vi "[CS] Main.vi"() -> ()   [LabVIEW 2014]
uses:
  NI Vision Camera Device/NI Vision Camera Device.lvclass
  NI Vision Camera Device/Configuration.ctl
panel:
  in  "Camera:Gain":dbl caption="Gain" min=0.0 max=20.0
  in  "Camera:Exposure":dbl=1000.0 caption="Exposure (µs)" min=20.0 max=1000000.0
  out "Camera":refnum<class "NI Vision Camera Device.lvclass">
  out "Camera:SizeY":u32=1040
  out "Camera:SizeX":u32=1392
  out "Avg":dbl[][](graph)
  out "Camera:FrameCount":u64
  out "Realtime":u16[][](graph)
  out "Exp:Progress":dbl(slide)=1.0 scale=0.0..1.0
  in  "Exp:MaxCount":u64=100
  in  "Exp:Start":bool
  in  "Exp:Cont":bool
  in  "Exp:Abort":bool
  in  "Camera:Threshold":u16=5 caption="Threshold"
  in  "Exp:Save":bool
  in  "Suffix":string
  in  "Camera:Start":bool
  in  "Camera:Stop":bool
  in  "Exp:Count":u64=100
  out "App:Basepath":path=path "C:/Users/mpdlab/Desktop/CameraSoftware/data"
  out "Camera:Sum":u64[][](array[numeric])
  out "App:Exit":bool
  out "Camera:Status":bool=TRUE
  # "Experiment"
  # "Camera"
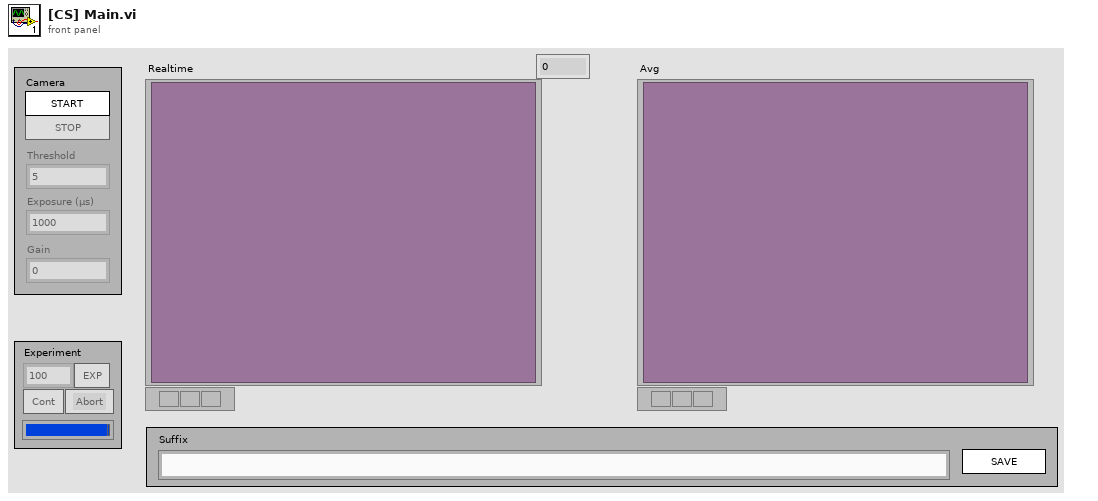
[diagram p1: front panel]
types:
  T1 = enum8{"Enabled", "Disabled", "Disabled and Grayed Out"}
  T2 = enum32{"invalid app kind", "Development System", "Run Time System", "Student Edition", "Embedded LabVIEW", "Evaluation", "Custom"}
  T3 = enum32{"Invalid", "Standard", "Closed", "Hidden", "Minimized", "Maximized"}
  T4 = typedef "NI Vision Camera Device.lvclass/Configuration.ctl" = cluster{"Exposure":dbl, "Gain":dbl}
  T5 = cluster{"Core":cluster{"Current VI Reference":refnum<vi>, "Close Panel on Exit?":bool}, "Camera:Status":bool}
  T6 = cluster{"Current VI Reference":refnum<vi>, "Close Panel on Exit?":bool}
  T7 = typedef "imagedata.ctl" = cluster{"image type":i32, "image depth":i32, "image":u8[], "mask":u8[], "colors":u32[], "Rectangle":cluster{"left":i16, "top":i16, "right":i16, "bottom":i16}}
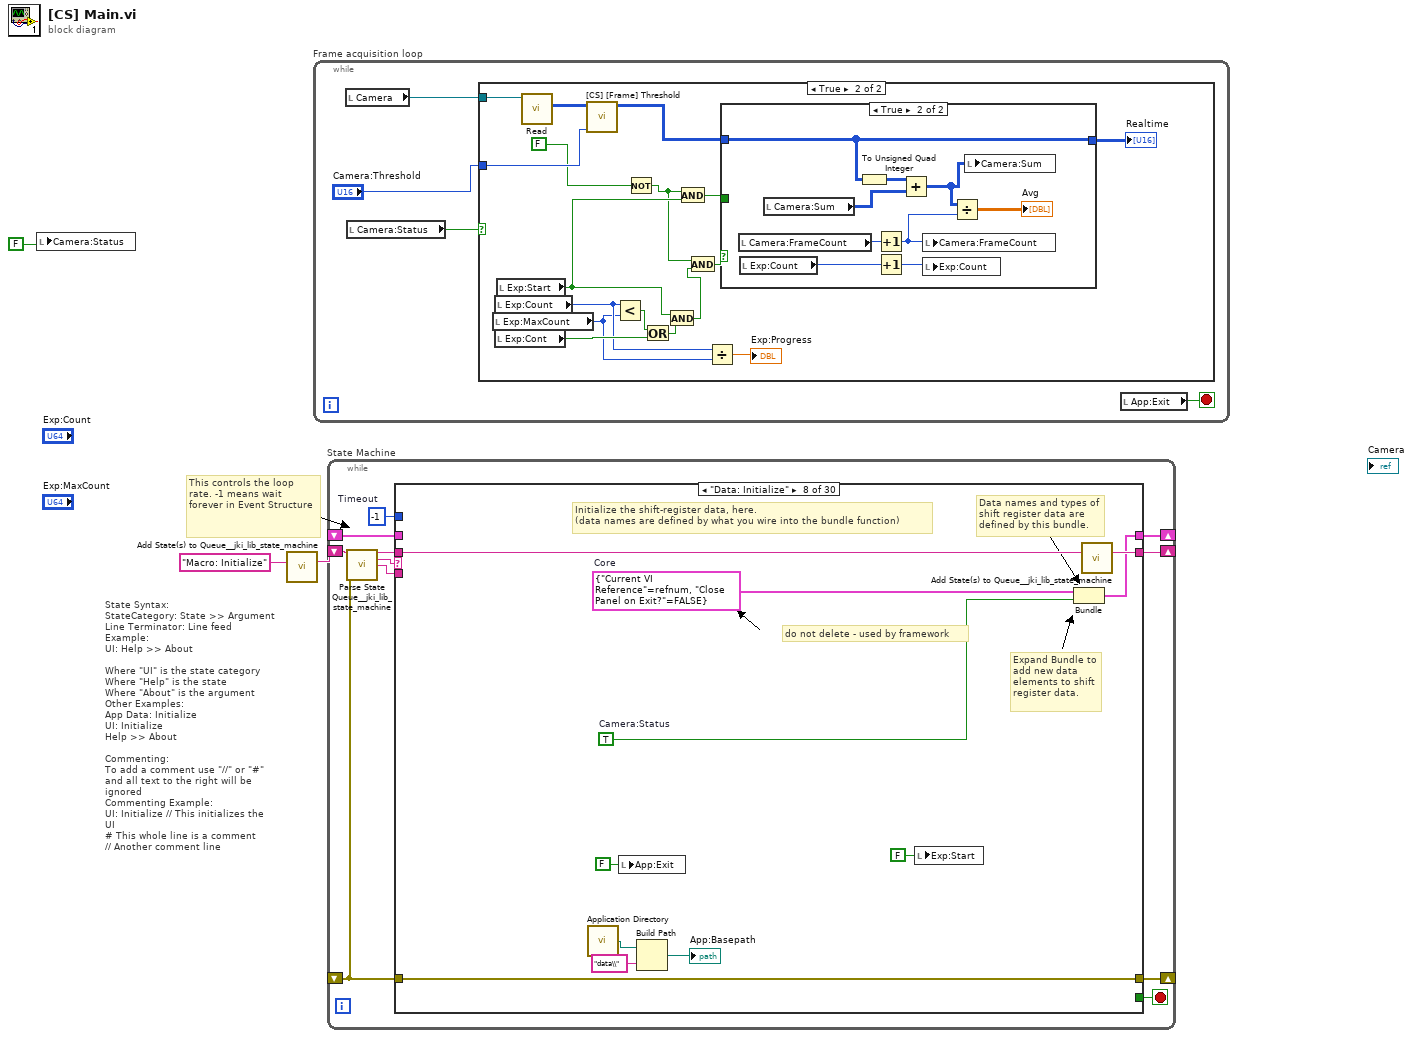
[diagram p0: block diagram]
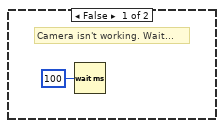
[diagram p2: hidden frame]
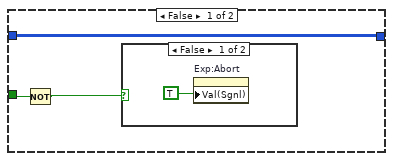
[diagram p3: hidden frame]
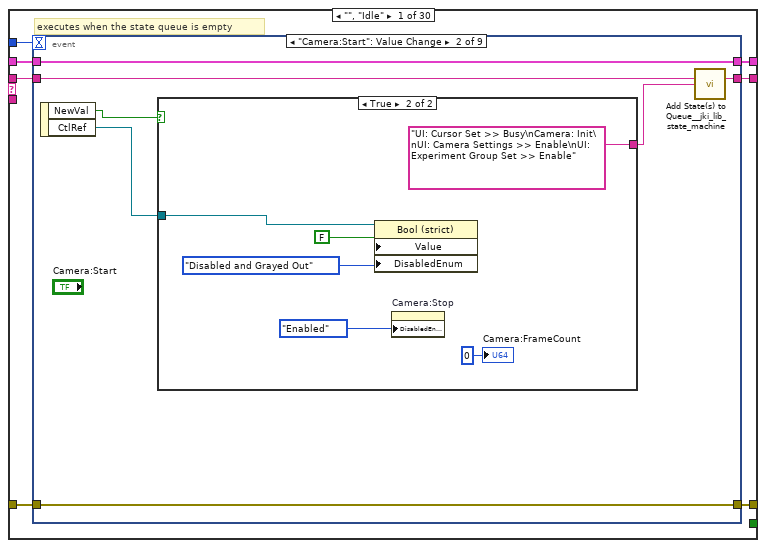
[diagram p5: hidden frame]
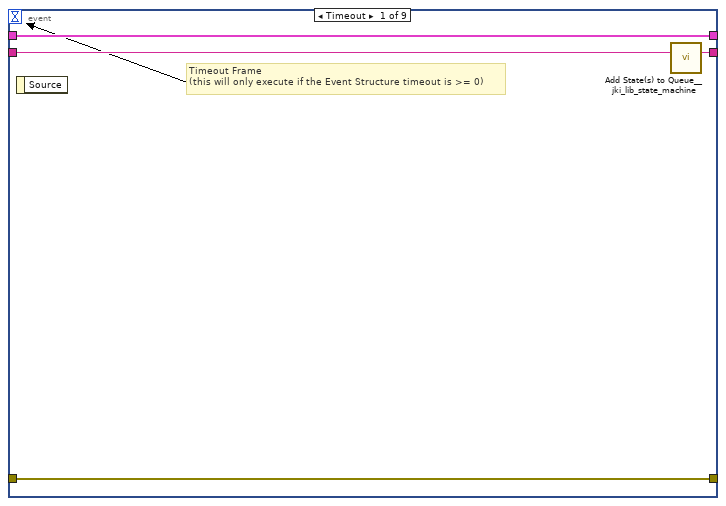
[diagram p6: hidden frame]
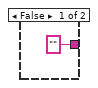
[diagram p7: hidden frame]
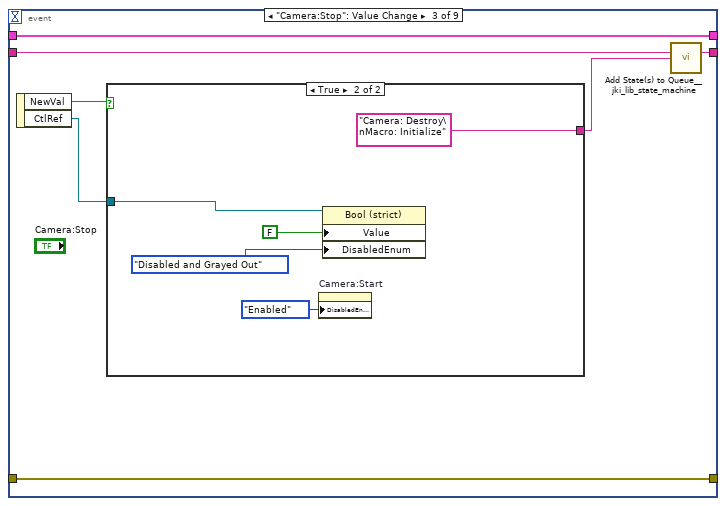
[diagram p8: hidden frame]
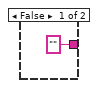
[diagram p9: hidden frame]
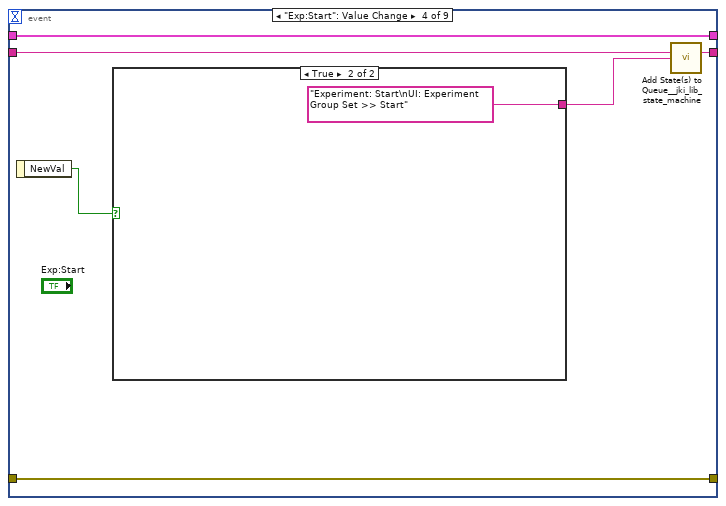
[diagram p10: hidden frame]
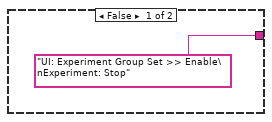
[diagram p11: hidden frame]
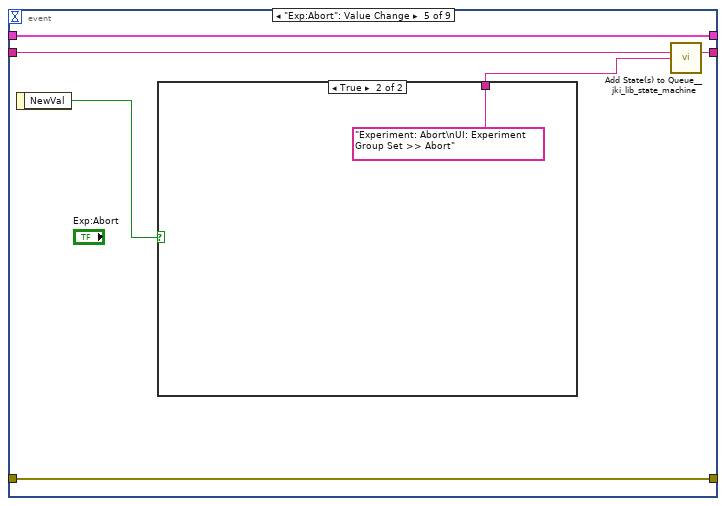
[diagram p12: hidden frame]
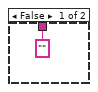
[diagram p13: hidden frame]
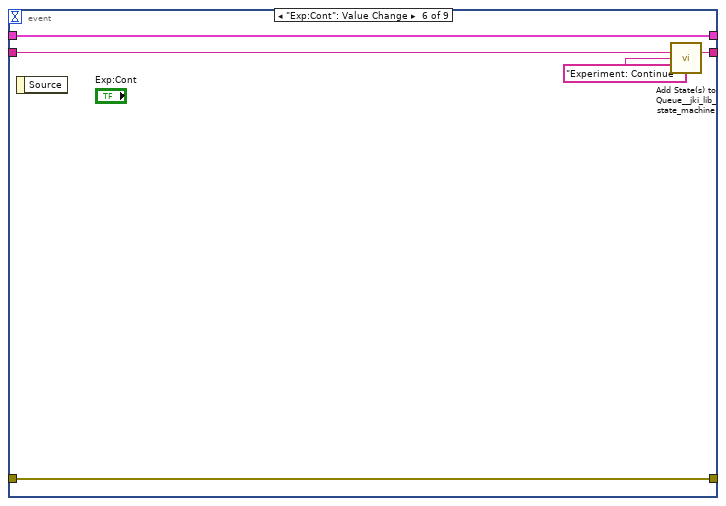
[diagram p14: hidden frame]
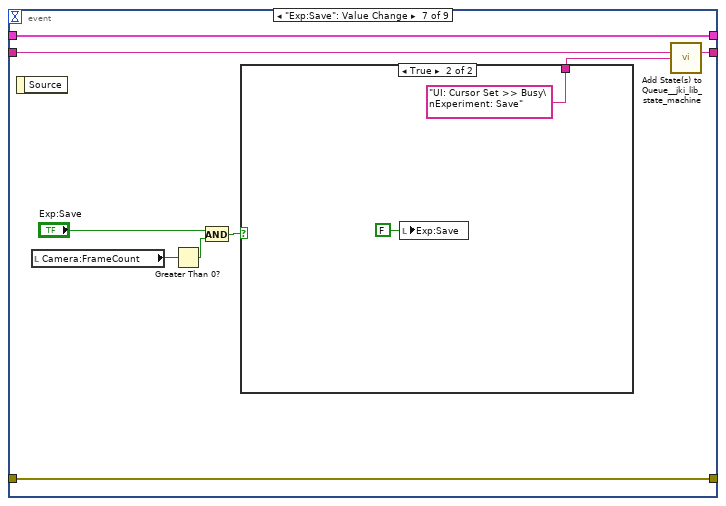
[diagram p15: hidden frame]
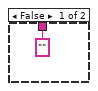
[diagram p16: hidden frame]
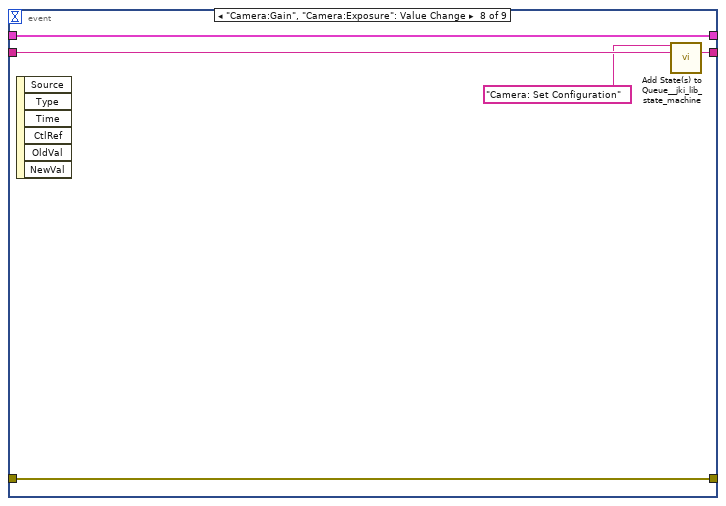
[diagram p17: hidden frame]
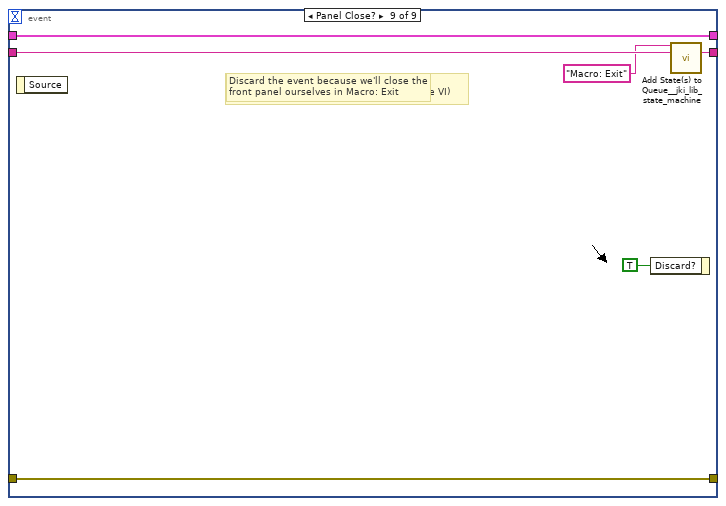
[diagram p18: hidden frame]
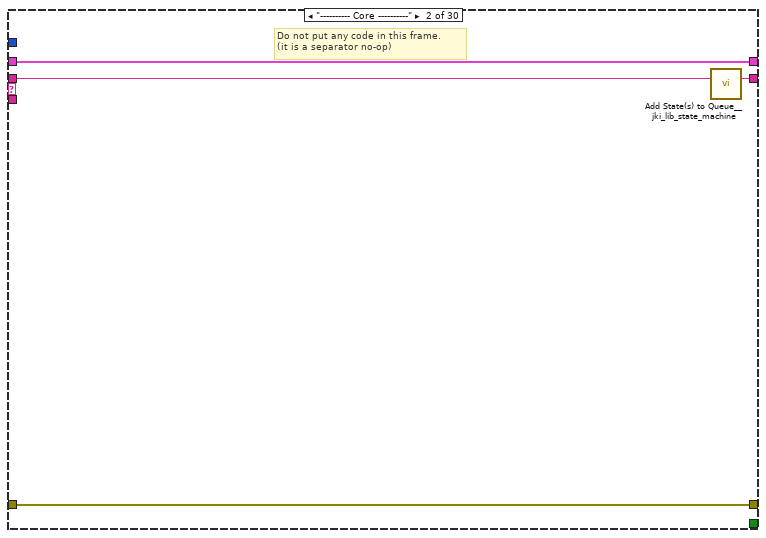
[diagram p19: hidden frame]
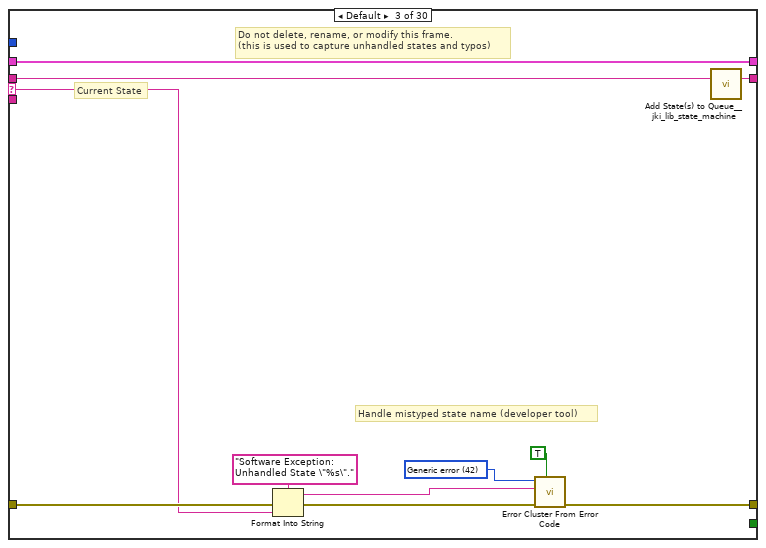
[diagram p20: hidden frame]
diagram:
  # "State Syntax:\nStateCategory: State >> Argument\nLine Terminator: Line feed\nExample:\nUI: Help >> About\n\nWhere \"UI\" is the state category\nWhere \"Help\" is the state\nWhere \"About\" is the argument\nOther Examples:\nApp Data: Initialize\nUI: Initialize\nHelp >> About\n\nCommenting:\nTo add a comment use \"//\" or \"#\" and all text to the right will be ignored\nCommenting Example:\nUI: Initialize // This initializes the UI\n# This whole line is a comment\n// Another comment line"
  # "This controls the loop rate. -1 means wait forever in Event Structure"
  n1 = local write "Camera:Status"(FALSE ("Camera:Status")) -> ()
  n2 = call <vilib>:"Add State(s) to Queue__jki_lib_state_machine.vi"("State(s) in (\"\")"="Macro: Initialize") -> ("States Out"=w3:string)  [unwired: 14 in]
  n3 = while "Frame acquisition loop" {
    stop <- w6 stop-if-true
    n4 = local read "Camera"() -> (w4:refnum<class "NI Vision Camera Device.lvclass">)
    n5 = local read "Camera:Status"() -> (w7:bool)
    n6 = case shown="True" w7 {
      tunnel: "Camera:Threshold" -> [_ w17]
      tunnel: w4 -> [_ w10]
      frame False {
        # "Camera isn't working. Wait..."
        n7 = Wait (ms)(milliseconds to wait=u32 100) -> ()  [unwired: 1 out]
      }
      frame True {
        n8 = local read "Exp:MaxCount"() -> (w22:u64)
        n9 = local read "Exp:Count"() -> (w23:u64)
        n10 = local read "Exp:Cont"() -> (w24:bool)
        n11 = local read "Exp:Start"() -> (w15:bool)
        n12 = call-dynamic "Read.vi"("NI Vision Camera Device in"=w10) -> ("Data"=w9:i16[][])  [unwired: 7 in, 3 out]
        n13 = call "[CS] [Frame] Threshold.vi"("Threshold"=w17, "buffer in"=w9) -> ("buffer out"=w18:u16[][])  [unwired: 9 in]
        n14 = Less?(x=w23, y=w22) -> (x < y?=w19:bool)
        n15 = Not(x=FALSE) -> (.not. x?=w12:bool)
        n16 = Or(x=w19, y=w24) -> (x .or. y?=w25:bool)
        n17 = And(x=w15, y=w25) -> (x .and. y?=w13:bool)
        n18 = And(x=w12, y=w15) -> (x .and. y?=w16:bool)
        n19 = And(x=w12, y=w13) -> (x .and. y?=w14:bool)
        n20 = Divide(x=w23, y=w22) -> (x/y=→"Exp:Progress":dbl)
        n21 = case shown="True" w14 {
          tunnel: [w28 w30] -> w20
          tunnel: w18 -> [w28 w30]
          tunnel: w16 -> [w27 _]
          frame False {
            n22 = Not(x=w27) -> (.not. x?=w26:bool)
            n23 = case shown="False" w26 {
              frame False {
                n24 = property on="Exp:Abort" class="Bool (strict)"("Val(Sgnl)"=TRUE ("Exp:Start")) -> ()  [unwired: 2 in, 2 out]
              }
              frame True {
              }
            }
          }
          frame True {
            n25 = local read "Camera:FrameCount"() -> (w38:u64)
            n26 = local read "Exp:Count"() -> (w32:u64)
            n27 = local read "Camera:Sum"() -> (w36:u64[][])
            n28 = To Unsigned Quad Integer(1:w30) -> (0:w35:u64[][])
            n29 = Increment(x=w38) -> (x+1=w37:u64)
            n30 = Increment(x=w32) -> (x+1=w33:u64)
            n31 = Add(x=w35, y=w36) -> (x+y=w34:u64[][])
            n32 = local write "Camera:FrameCount"(w37) -> ()
            n33 = local write "Exp:Count"(w33) -> ()
            n34 = Divide(x=w34, y=w37) -> (x/y=→"Avg":dbl[][])
            n35 = local write "Camera:Sum"(w34) -> ()
          }
        }
        "Realtime" <- w20
      }
    }
    n36 = local read "App:Exit"() -> (w6:bool)
  }
  n37 = while "State Machine" {
    shift-right: [w43] -> _
    shift-left: _ -> [w42]
    shift-right: [w45] -> _
    shift-left: _ -> [w40]
    shift-right: [w44] -> _
    shift-left: w3 -> [w46]
    stop <- w39 stop-if-true
    w41 = -1  # Timeout
    n38 = call <vilib>:"Parse State Queue__jki_lib_state_machine.vi"("State Queue"=w46, "Error In (no error)"=w40) -> ("Remaining States"=w48:string, "Current State"=w49:string, "Arguments"=w47:string)  [unwired: 11 in]
    n39 = case shown="\"Data: Initialize\"" w49 {
      selector: w49 -> [_ _ w136 _ _ _ _ _ _ _ _ _ _ _ _ _ _ _ _ _ _ _ _ _ _ _ _ _ _ _]
      tunnel: w48 -> [w56 w135 w140 w158 w164 w169 w173 w184 w190 w194 w203 w212 w224 w232 w243 w269 w274 w284 w288 w304 w315 w329 w337 w349 w353 w358 w364 w368 w389 w399]
      tunnel: w47 -> [_ _ _ _ _ _ _ _ _ _ _ w208 w220 w227 w237 _ _ _ _ _ _ _ _ _ _ _ _ _ _ _]
      tunnel: w42 -> [w54 w132 w138 w149 w161 w167 w170 _ w185 w191 w201 w210 w222 w230 w239 w266 w271 w281 w285 w295 w313 w327 w335 w346 w350 w355 w361 w365 w386 w396]
      tunnel: [w53 w133 w142 w155 errorcluster {"status"=FALSE, "code"=0, "source"=""} ("error out") w166 w171 w181 w186 w192 w200 w209 w221 w228 w240 w267 w272 w282 w286 w289 w310 w326 w332 w347 w351 w356 w362 w366 w387 w397] -> w45
      tunnel: w40 -> [w52 w133 w141 w155 w160 w166 w171 w181 w187 w192 w200 w209 w221 w229 w241 w267 w272 w282 w286 w294 w310 w326 w333 w347 w351 w356 w362 w366 w387 w397]
      tunnel: [w55 w134 w139 w157 w163 w168 w172 w183 w189 w193 w202 w211 w223 w231 w242 w268 w273 w283 w287 w303 w314 w328 w336 w348 w352 w357 w363 w367 w388 w398] -> w44
      tunnel: [_ _ _ _ _ w165 _ _ _ _ _ _ _ _ _ _ _ _ _ _ _ _ _ _ _ _ _ _ _ _] -> w39
      tunnel: [w51 w132 w138 w156 w161 w167 w170 w182 w185 w191 w201 w210 w222 w230 w239 w266 w271 w281 w285 w295 w313 w327 w335 w346 w350 w355 w361 w365 w386 w396] -> w43
      tunnel: w41 -> [w50 _ _ _ _ _ _ _ _ _ _ _ _ _ _ _ _ _ _ _ _ _ _ _ _ _ _ _ _ _]
      frame "", "Idle" {
        # "executes when the state queue is empty"
        n40 = event shown="[1] \"Camera:Start\": Value Change" {
          selector: _ -> [_ _ _ _ _ _ _ _ _]
          dyn-events: _ -> [_ _ _ _ _ _ _ _ _]
          timeout: w50 -> [_ _ _ _ _ _ _ _ _]
          tunnel: w56 -> [w60 w67 w81 w93 w101 w108 w117 w125 w131]
          tunnel: [w59 w66 w80 w92 w100 w107 w116 w124 w130] -> w55
          tunnel: w54 -> [w57 w64 w78 w90 w98 w105 w114 w123 w128]
          tunnel: [w58 w65 w79 w91 w99 w106 w115 w122 w129] -> w53
          tunnel: w52 -> [w58 w65 w79 w91 w99 w106 w115 w122 w129]
          tunnel: [w57 w64 w78 w90 w98 w105 w114 w123 w128] -> w51
          event Timeout {
            # "Timeout Frame\n(this will only execute if the Event Structure timeout is >= 0)"
            n41 = event-data() -> ()  [unwired: 1 in, 1 out]
            n42 = call <vilib>:"Add State(s) to Queue__jki_lib_state_machine.vi"("State(s) in (\"\")"=w60) -> ("States Out"=w59:string)  [unwired: 14 in]
          }
          event "Camera:Start": Value Change {
            n43 = event-data() -> ("NewVal"=w63:bool, "CtlRef"=w61:refnum<vi>)  [unwired: 1 in]
            n44 = case shown="True" w63 {
              tunnel: ["" "UI: Cursor Set >> Busy\nCamera: Init\nUI: Camera Settings >> Enable\nUI: Experiment Group Set >> Enable"] -> w62
              tunnel: w61 -> [_ w73]
              frame False {
              }
              frame True {
                n45 = property class="Bool (strict)"(reference=w73, "Value"=FALSE, "DisabledEnum"=T1."Disabled and Grayed Out" ("Disabled")) -> ()  [unwired: 1 in, 2 out]
                n46 = property on="Camera:Stop" class="Bool (strict)"("DisabledEnum"=T1."Enabled" ("Disabled")) -> ()  [unwired: 2 in, 2 out]
                "Camera:FrameCount" <- u64 0 ("Camera:FrameCount")
              }
            }
            n47 = call <vilib>:"Add State(s) to Queue__jki_lib_state_machine.vi"("State(s) in (\"\")"=w67, "State(s) at Back (\"\")"=w62) -> ("States Out"=w66:string)  [unwired: 13 in]
          }
          event "Camera:Stop": Value Change {
            n48 = event-data() -> ("NewVal"=w77:bool, "CtlRef"=w76:refnum<vi>)  [unwired: 1 in]
            n49 = case shown="True" w77 {
              tunnel: ["" "Camera: Destroy\nMacro: Initialize"] -> w75
              tunnel: w76 -> [_ w86]
              frame False {
              }
              frame True {
                n50 = property on="Camera:Start" class="Bool (strict)"("DisabledEnum"=T1."Enabled" ("Disabled")) -> ()  [unwired: 2 in, 2 out]
                n51 = property class="Bool (strict)"(reference=w86, "Value"=FALSE, "DisabledEnum"=T1."Disabled and Grayed Out" ("Disabled")) -> ()  [unwired: 1 in, 2 out]
              }
            }
            n52 = call <vilib>:"Add State(s) to Queue__jki_lib_state_machine.vi"("State(s) in (\"\")"=w81, "State(s) at Back (\"\")"=w75) -> ("States Out"=w80:string)  [unwired: 13 in]
          }
          event "Exp:Start": Value Change {
            n53 = event-data() -> ("NewVal"=w89:bool)  [unwired: 1 in]
            n54 = case shown="True" w89 {
              tunnel: ["UI: Experiment Group Set >> Enable\nExperiment: Stop" "Experiment: Start\nUI: Experiment Group Set >> Start"] -> w88
              frame False {
              }
              frame True {
              }
            }
            n55 = call <vilib>:"Add State(s) to Queue__jki_lib_state_machine.vi"("State(s) in (\"\")"=w93, "State(s) at Back (\"\")"=w88) -> ("States Out"=w92:string)  [unwired: 13 in]
          }
          event "Exp:Abort": Value Change {
            n56 = event-data() -> ("NewVal"=w96:bool)  [unwired: 1 in]
            n57 = case shown="True" w96 {
              tunnel: ["" "Experiment: Abort\nUI: Experiment Group Set >> Abort"] -> w97
              frame False {
              }
              frame True {
              }
            }
            n58 = call <vilib>:"Add State(s) to Queue__jki_lib_state_machine.vi"("State(s) in (\"\")"=w101, "State(s) at Back (\"\")"=w97) -> ("States Out"=w100:string)  [unwired: 13 in]
          }
          event "Exp:Cont": Value Change {
            n59 = event-data() -> ()  [unwired: 1 in, 1 out]
            n60 = call <vilib>:"Add State(s) to Queue__jki_lib_state_machine.vi"("State(s) in (\"\")"=w108, "State(s) at Back (\"\")"="Experiment: Continue") -> ("States Out"=w107:string)  [unwired: 13 in]
          }
          event "Exp:Save": Value Change {
            n61 = event-data() -> ()  [unwired: 1 in, 1 out]
            n62 = local read "Camera:FrameCount"() -> (w112:u64)
            n63 = Greater Than 0?(x=w112) -> (x > 0?=w111:bool)
            n64 = And(x="Exp:Save", y=w111) -> (x .and. y?=w110:bool)
            n65 = case shown="True" w110 {
              tunnel: ["" "UI: Cursor Set >> Busy\nExperiment: Save"] -> w113
              frame False {
              }
              frame True {
                n66 = local write "Exp:Save"(FALSE ("Exp:Save")) -> ()
              }
            }
            n67 = call <vilib>:"Add State(s) to Queue__jki_lib_state_machine.vi"("State(s) in (\"\")"=w117, "State(s) at Back (\"\")"=w113) -> ("States Out"=w116:string)  [unwired: 13 in]
          }
          event "Camera:Gain", "Camera:Exposure": Value Change {
            n68 = event-data() -> ()  [unwired: 1 in, 6 out]
            n69 = call <vilib>:"Add State(s) to Queue__jki_lib_state_machine.vi"("State(s) in Front (\"\")"="Camera: Set Configuration" ("State(s) in Front (\"\")"), "State(s) in (\"\")"=w125) -> ("States Out"=w124:string)  [unwired: 13 in]
          }
          event Panel Close? {
            # "Discard the event because we'll close the front panel ourselves in Macro: Exit"
            # "Close Panel button (pressed) Event\n(this executes Macro: Exit to terminate the VI)"
            n70 = event-data() -> ()  [unwired: 1 in, 1 out]
            n71 = event-data("Discard?"=TRUE) -> ()  [unwired: 1 in, 1 out]
            n72 = call <vilib>:"Add State(s) to Queue__jki_lib_state_machine.vi"("State(s) in Front (\"\")"="Macro: Exit", "State(s) in (\"\")"=w131) -> ("States Out"=w130:string)  [unwired: 13 in]
          }
        }
      }
      frame "---------- Core ----------" {
        # "Do not put any code in this frame.\n(it is a separator no-op)"
        n73 = call <vilib>:"Add State(s) to Queue__jki_lib_state_machine.vi"("State(s) in (\"\")"=w135) -> ("States Out"=w134:string)  [unwired: 14 in]
      }
      frame Default {
        w145 = 42 items=["No error", "Argument error", "Memory is full", "Out of zone", "End of file", "File already open", "Generic file I/O error", "File not found", "File permission error", "Disk is full", "Duplicate path", "Too many files open", "System feature not enabled", "Resource file not found", "Cannot add resource", "Resource not found", "Image not found", "Image memory error", "Pen does not exist", "Config type invalid", "Config token not found", "Config parse error", "Config memory error", "Bad external code format", "Bad external code offset", "External code not present", "Null window", "Destroy window error", "Null menu", "Print aborted", "Bad print record", "Print driver error", "Windows error during printing", "Memory error during printing", "Print dialog error", "Generic print error", "Invalid device refnum", "Device not found", "Device parameter error", "Device unit error", "Cannot open device", "Device call aborted", "Generic error", "Cancelled by user", "Object ID too low", "Object ID too high", "Object not in heap", "Unknown heap", "Unknown object (invalid DefProc)", "Unknown object (DefProc not in table)", "Message out of range", "Invalid (null) method", "Unknown message", "Manager call not supported", "Bad address", "Network operation in progress", "Network operation timed out", "Connection is busy", "Network attribute not supported", "Network error", "Address in use", "System out of memory", "Connection aborted", "Connection refused", "Not connected", "Already connected", "Connection closed", "Initialization error (interapplication manager)", "Bad occurrence", "Wait on unbound occurrence handler", "Occurrence queue overflow", "Datalog type conflict", "Unused", "Unrecognized type (interapplication manager)", "Memory corrupt", "Failed to make temporary DLL", "Old CIN version", "Drag socket not found", "Failed to load drop-object", "Failed to register OLE object", "Failed to release OLE object", "Format specifier type mismatch", "Unknown format specifier", "Too few format specifiers", "Too many format specifiers", "Scan failed", "Newer CIN version", "Error converting to variant", "Runtime menu error", "Password tampered", "Variant attribute not found", "Incompatible variant data type", "Event data is not available", "Event Store is not present", "Occurrence is not found", "Event Queue is not created", "Event info is not available", "Refnum passed is NULL", "Error retrieving Class GUID", "Error retrieving CoClass GUID", "Error retrieving TypeLib GUID.", "Bad built application magic bytes.", "Specific driver is different from the specific driver associated with the Logical Name.", "There is no session opened to the class driver.", "Max Error", "MAX - Error with config objects", "MAX - Error loading configuration", "MAX - Group not supported"]
        # "Current State"
        # "Do not delete, rename, or modify this frame.\n(this is used to capture unhandled states and typos)"
        # "Handle mistyped state name (developer tool)"
        n74 = Format Into String(format string="Software Exception: Unhandled State \"%s\"." ("message"), error in=w141, w136) -> (resulting string=w144:string, error out=w143:errorcluster)  [unwired: 1 in]
        n75 = call <vilib>:"Error Cluster From Error Code.vi"("show call chain? (False)"=TRUE, "error in (no error)"=w143, "error message (\"\")"=w144, "error code (0)"=w145) -> ("error out"=w142:errorcluster)  [unwired: 5 in]
        n76 = call <vilib>:"Add State(s) to Queue__jki_lib_state_machine.vi"("State(s) in (\"\")"=w140) -> ("States Out"=w139:string)  [unwired: 14 in]
      }
      frame "Initialize Core Data" {
        # "Do not delete, rename, or modify this frame.\n(this is used to determine panel behavior on exit)"
        # "originally closed?"
        # "exe?"
        # "If panel starts closed or is an EXE, then close it when we exit"
        n77 = property class="VI"() -> ("Front Panel.Open"=w154:bool)  [unwired: 2 in, 2 out]
        n78 = property class="App"() -> ("App.Kind"=w153:T2)  [unwired: 2 in, 2 out]
        n79 = control-ref of="Current VI Reference"() -> (w147:refnum<vi>)
        n80 = Not(x=w154) -> (.not. x?=w151:bool)
        n81 = Equal?(x=w153, y=T2."Run Time System" ("Application:Kind")) -> (x = y?=w150:bool)
        n82 = Or(x=w151, y=w150) -> (x .or. y?=w148:bool)
        n83 = Bundle By Name(cluster=w149, "Core.Current VI Reference"=w147, "Core.Close Panel on Exit?"=w148) -> (w156:T5)
        n84 = call <vilib>:"Add State(s) to Queue__jki_lib_state_machine.vi"("State(s) in (\"\")"=w158) -> ("States Out"=w157:string)  [unwired: 14 in]
      }
      frame "Error Handler" {
        # "Unhandled Error -- Display it"
        # "Handle any errors here.\nYou can also output any states to clean-up after errors occur"
        # "Clear error"
        n85 = call <vilib>:"General Error Handler.vi"("error in (no error)"=w160) -> ()  [unwired: 10 in, 5 out]
        n86 = call <vilib>:"Add State(s) to Queue__jki_lib_state_machine.vi"("State(s) in Front (\"\")"="/* Post Error States", "State(s) in (\"\")"=w164) -> ("States Out"=w163:string)  [unwired: 13 in]
      }
      frame "Exit" {
        w165 = TRUE
        # "Do not put any code in this frame.\n(No errors that occur here will be handled.)"
        n87 = call <vilib>:"Add State(s) to Queue__jki_lib_state_machine.vi"("State(s) in (\"\")"=w169) -> ("States Out"=w168:string)  [unwired: 14 in]
        "App:Exit" <- w165
      }
      frame "---------- Data ----------" {
        # "Do not put any code in this frame.\n(It is a separator no-op. You can make a copy of this frame to create a new Data frame)"
        n88 = call <vilib>:"Add State(s) to Queue__jki_lib_state_machine.vi"("State(s) in (\"\")"=w173) -> ("States Out"=w172:string)  [unwired: 14 in]
      }
      frame "Data: Initialize" {
        w179 = T6 {"Current VI Reference"=refnum, "Close Panel on Exit?"=FALSE}  # Core
        w180 = TRUE  # Camera:Status
        # "do not delete - used by framework"
        # "Expand Bundle to add new data elements to shift register data."
        # "Data names and types of shift register data are defined by this bundle."
        # "Initialize the shift-register data, here.\n(data names are defined by what you wire into the bundle function)"
        n89 = call <vilib>:"Application Directory.vi"() -> ("Application Directory"=w176:path)
        n90 = local write "App:Exit"(FALSE ("App:Exit")) -> ()
        n91 = Build Path(base path=w176, name or relative path="data\\") -> (appended path=→"App:Basepath":path)
        n92 = local write "Exp:Start"(FALSE ("Exp:Start")) -> ()
        n93 = Bundle("Core"=w179, "Camera:Status"=w180) -> (w182:T5)  [unwired: 1 in]
        n94 = call <vilib>:"Add State(s) to Queue__jki_lib_state_machine.vi"("State(s) in (\"\")"=w184) -> ("States Out"=w183:string)  [unwired: 14 in]
      }
      frame "Data: Cleanup" {
        # "Cleanup any data and references, here.\n(this is called automatically, by the Macro: Exit)"
        n95 = Unbundle By Name(w185) -> ("Core.Current VI Reference"=w188:refnum<vi>)
        n96 = Close Reference(reference=w188, error in (no error)=w187) -> (error out=w186:errorcluster)
        n97 = call <vilib>:"Add State(s) to Queue__jki_lib_state_machine.vi"("State(s) in (\"\")"=w190) -> ("States Out"=w189:string)  [unwired: 14 in]
      }
      frame "---------- UI ----------" {
        # "Do not put any code in this frame.\n(It is a separator no-op. You can make a copy of this frame to create a new UI frame)"
        n98 = call <vilib>:"Add State(s) to Queue__jki_lib_state_machine.vi"("State(s) in (\"\")"=w194) -> ("States Out"=w193:string)  [unwired: 14 in]
      }
      frame "UI: Initialize" {
        # "Initialize the User Interface, here.\n(this is called automatically, by the Macro: Init)"
        n99 = property on="Camera:Stop" class="Bool (strict)"("DisabledEnum"=T1."Disabled and Grayed Out" ("Disabled"), "Value"=FALSE ("Camera:Stop")) -> ()  [unwired: 2 in, 2 out]
        n100 = property on="Camera:Start" class="Bool (strict)"("DisabledEnum"=T1."Enabled" ("Disabled"), "Value"=FALSE ("Camera:Start")) -> ()  [unwired: 2 in, 2 out]
        n101 = call <vilib>:"Add State(s) to Queue__jki_lib_state_machine.vi"("State(s) in (\"\")"=w203, "State(s) at Back (\"\")"="UI: Camera Settings >> Disable\nUI: Experiment Group Set >> Disable" ("State(s) at Back (\"\")")) -> ("States Out"=w202:string)  [unwired: 13 in]
      }
      frame "UI: Experiment Group Set" {
        # "Initialize the User Interface, here.\n(this is called automatically, by the Macro: Init)"
        n102 = case shown="\"Abort\", \"Init\", Default" w208 {
          tunnel: [T1."Disabled and Grayed Out" ("Disabled") w216 T1."Enabled" ("Disabled")] -> w205
          tunnel: [T1."Enabled" ("Disabled") w216 T1."Disabled and Grayed Out" ("Disabled")] -> w204
          frame "Abort", "Init", Default {
            n103 = local write "Exp:Start"(FALSE ("Exp:Start")) -> ()
          }
          frame "Disable" {
            w216 = T1."Disabled and Grayed Out" ("Disabled")
          }
          frame "Start" {
          }
        }
        n104 = property on="Exp:Start" class="Bool (strict)"("DisabledEnum"=w204) -> ()  [unwired: 2 in, 2 out]
        n105 = property on="Exp:Cont" class="Bool (strict)"("DisabledEnum"=w205, "Value"=FALSE ("Exp:Cont")) -> ()  [unwired: 2 in, 2 out]
        n106 = property on="Exp:MaxCount" class="DigNum (strict)"("DisabledEnum"=w204) -> ()  [unwired: 2 in, 2 out]
        n107 = property on="Exp:Abort" class="Bool (strict)"("DisabledEnum"=w205, "Value"=FALSE ("Exp:Abort")) -> ()  [unwired: 2 in, 2 out]
        n108 = call <vilib>:"Add State(s) to Queue__jki_lib_state_machine.vi"("State(s) in (\"\")"=w212) -> ("States Out"=w211:string)  [unwired: 14 in]
      }
      frame "UI: Camera Settings" {
        # "Initialize the User Interface, here.\n(this is called automatically, by the Macro: Init)"
        n109 = case shown="\"Enable\"" w220 {
          tunnel: [T1."Disabled and Grayed Out" ("Disabled") T1."Enabled" ("Disabled")] -> w219
          frame "Disable", Default {
          }
          frame "Enable" {
          }
        }
        n110 = property on="Camera:Threshold" class="DigNum (strict)"("DisabledEnum"=w219) -> ()  [unwired: 2 in, 2 out]
        n111 = property on="Camera:Exposure" class="DigNum (strict)"("DisabledEnum"=w219) -> ()  [unwired: 2 in, 2 out]
        n112 = property on="Camera:Gain" class="DigNum (strict)"("DisabledEnum"=w219) -> ()  [unwired: 2 in, 2 out]
        n113 = call <vilib>:"Add State(s) to Queue__jki_lib_state_machine.vi"("State(s) in (\"\")"=w224) -> ("States Out"=w223:string)  [unwired: 14 in]
      }
      frame "UI: Cursor Set" {
        # "Argument"
        # "Set and Unset Cursor Busy.\n(Usage: \"UI: Cursor Set >> Busy|Idle\")"
        n114 = case shown="\"Busy\"" w227 {
          tunnel: w229 -> [w234 w236]
          tunnel: [w233 w235] -> w228
          frame "Idle", Default {
            n115 = call <vilib>:"Unset Busy.vi"("error in (no error)"=w234) -> ("error out"=w233:errorcluster)  [unwired: 10 in]
          }
          frame "Busy" {
            n116 = call <vilib>:"Set Busy.vi"("error in (no error)"=w236) -> ("error out"=w235:errorcluster)  [unwired: 9 in, 1 out]
          }
        }
        n117 = call <vilib>:"Add State(s) to Queue__jki_lib_state_machine.vi"("State(s) in (\"\")"=w232) -> ("States Out"=w231:string)  [unwired: 14 in]
      }
      frame "UI: Front Panel State" {
        # "Argument"
        # "Set Front Panel Open or Closed\n(Usage: \"UI: Front Panel State >> Open|Close\")"
        n118 = Unbundle By Name(w239) -> ("Core.Current VI Reference"=w238:refnum<vi>)
        n119 = case shown="\"Open\", Default" w237 {
          tunnel: w241 -> [w247 w260]
          tunnel: [w249 w261] -> w240
          tunnel: w238 -> [w248 w258]
          frame "Open", Default {
            n120 = property class="VI"(reference=w248, error in=w247) -> (reference out=w245:refnum<vi>, error out=w246:errorcluster, "Front Panel.Open"=w244:bool)
            n121 = case shown="False" w244 {
              tunnel: [w252 w255] -> w249
              tunnel: w246 -> [w251 w255]
              tunnel: w245 -> [w250 _]
              frame False {
                n122 = invoke class="VI" method="FP.Open"(reference=w250, error in=w251, "Activate"=TRUE, "State"=T3."Standard") -> (error out=w252:errorcluster)  [unwired: 1 in, 4 out]
              }
              frame True {
              }
            }
          }
          frame "Close" {
            n123 = property class="VI"(reference=w258, error in=w260) -> (reference out=w257:refnum<vi>, error out=w259:errorcluster, "Front Panel.Open"=w256:bool)
            n124 = case shown="True" w256 {
              tunnel: [w262 w265] -> w261
              tunnel: w259 -> [w262 w264]
              tunnel: w257 -> [_ w263]
              frame False {
              }
              frame True {
                n125 = invoke class="VI" method="FP.Close"(reference=w263, error in=w264) -> (error out=w265:errorcluster)  [unwired: 1 in, 2 out]
              }
            }
          }
        }
        n126 = call <vilib>:"Add State(s) to Queue__jki_lib_state_machine.vi"("State(s) in (\"\")"=w243) -> ("States Out"=w242:string)  [unwired: 14 in]
      }
      frame "---------- Macro ----------" {
        # "Do not put any code in this frame.\n(It is a separator no-op. You can make a copy of this frame to create a new Macro frame)"
        n127 = call <vilib>:"Add State(s) to Queue__jki_lib_state_machine.vi"("State(s) in (\"\")"=w269) -> ("States Out"=w268:string)  [unwired: 14 in]
      }
      frame "Macro: Initialize" {
        w270 = "Data: Initialize\nInitialize Core Data\nUI: Initialize\nUI: Front Panel State >> Open"  # Data: Initialize Initialize Core Data UI: Initialize UI: Front Panel State >> Open
        # "Initialization Macro\n(This is called once, when the VI starts)"
        n128 = call <vilib>:"Add State(s) to Queue__jki_lib_state_machine.vi"("State(s) in Front (\"\")"=w270, "State(s) in (\"\")"=w274) -> ("States Out"=w273:string)  [unwired: 13 in]
      }
      frame "Macro: Exit" {
        # "Exit Macro\n(This is called once, when the VI exits)"
        n129 = Unbundle By Name(w281) -> ("Core.Close Panel on Exit?"=w280:bool)
        n130 = Select(t="UI: Front Panel State >> Close", s=w280, f="") -> (s? t:f=w277:string)
        n131 = call <vilib>:"Add State(s) to Queue__jki_lib_state_machine.vi"("State(s) in (\"\")"=w277, "State(s) at Back (\"\")"="Data: Cleanup\nExit") -> ("States Out"=w275:string)  [unwired: 13 in]
        n132 = call <vilib>:"Add State(s) to Queue__jki_lib_state_machine.vi"("State(s) in Front (\"\")"=w275, "State(s) in (\"\")"=w284) -> ("States Out"=w283:string)  [unwired: 13 in]
      }
      frame "---------- VS Camera ----------" {
        # "Template Separator\n(You can make a copy of, or modify, this frame)"
        n133 = call <vilib>:"Add State(s) to Queue__jki_lib_state_machine.vi"("State(s) in (\"\")"=w288) -> ("States Out"=w287:string)  [unwired: 14 in]
      }
      frame "Camera: Init" {
        w293 = refnum<class "NI Vision Camera Device.lvclass"> refnum  # NI Vision Camera Device.lvclass
        w296 = u32 1536
        w297 = u32 2048
        n134 = call-dynamic "Connect.vi"("error in (no error)"=w294, "NI Vision Camera Device in"=w293) -> ("error out"=w290:errorcluster, "NI Vision Camera Device out"=w292:refnum<class "NI Vision Camera Device.lvclass">)  [unwired: 8 in]
        n135 = property on="Realtime" class="IntGraph (strict)"("XScale.Minimum"=0.0 ("X Scale.Range:Minimum"), "XScale.Maximum"=w297, "YScale.Minimum"=0.0 ("Y Scale.Range:Minimum"), "YScale.Maximum"=w296) -> ()  [unwired: 2 in, 2 out]
        n136 = property on="Avg" class="IntGraph (strict)"("XScale.Minimum"=0.0 ("X Scale.Range:Minimum"), "XScale.Maximum"=w297, "YScale.Minimum"=0.0 ("Y Scale.Range:Minimum"), "YScale.Maximum"=w296) -> ()  [unwired: 2 in, 2 out]
        n137 = local write "Camera"(w292) -> ()
        n138 = property on="Camera:Status" class="Bool (strict)"(error in=w290, "Val(Sgnl)"=TRUE ("Value (Signaling)")) -> (error out=w289:errorcluster)  [unwired: 1 in, 1 out]
        n139 = call <vilib>:"Add State(s) to Queue__jki_lib_state_machine.vi"("State(s) in (\"\")"=w304, "State(s) at Back (\"\")"="UI: Cursor Set >> Idle\nCamera: Config" ("State(s) at Back (\"\")")) -> ("States Out"=w303:string)  [unwired: 13 in]
        "Camera:SizeX" <- w297
        "Camera:SizeY" <- w296
      }
      frame "Camera: Config" {
        # "Your code here.\n(You can make a copy of, or modify, this frame)"
        n140 = property on="Camera:Gain" class="DigNum (strict)"("Value"=0.0 ("Camera:Gain")) -> ()  [unwired: 2 in, 2 out]
        n141 = property on="Camera:Exposure" class="DigNum (strict)"("Value"=1000.0 ("Camera:Exposure")) -> ()  [unwired: 2 in, 2 out]
        n142 = local read "Camera:SizeY"() -> (w309:u32)
        n143 = local read "Camera:SizeX"() -> (w308:u32)
        n144 = Initialize Array(u64 0 ("element"), w309, w308) -> (w311:u64[][])
        "Camera:Sum" <- w311
        n145 = local write "Avg"(w311) -> ()
        n146 = local write "Realtime"(w311) -> ()
        n147 = call <vilib>:"Add State(s) to Queue__jki_lib_state_machine.vi"("State(s) in Front (\"\")"="Camera: Set Configuration" ("State(s) in Front (\"\")"), "State(s) in (\"\")"=w315) -> ("States Out"=w314:string)  [unwired: 13 in]
      }
      frame "Camera: Set Configuration" {
        # "Your code here.\n(You can make a copy of, or modify, this frame)"
        n148 = local read "Camera"() -> (w323:refnum<class "NI Vision Camera Device.lvclass">)
        n149 = Bundle By Name(cluster=T4 {"Exposure"=0.0, "Gain"=0.0} ("Configuration"), "Exposure"="Camera:Exposure", "Gain"="Camera:Gain") -> (w321:T4)
        n150 = call "Set Camera Configuration.vi"("Configuration"=w321, "NI Vision Camera in"=w323) -> ("error out"=w325:errorcluster, "NI Vision Camera out"=w324:refnum<class "NI Vision Camera Device.lvclass">)  [unwired: 8 in]
        n151 = call "Get Camera Configuration.vi"("error in (no error)"=w325, "NI Vision Camera Device in"=w324) -> ("Configuration"=w320:T4)  [unwired: 7 in, 2 out]
        n152 = Unbundle By Name(w320) -> ("Exposure"=w319:dbl, "Gain"=w318:dbl)
        n153 = property on="Camera:Gain" class="DigNum (strict)"("Value"=w318) -> ()  [unwired: 2 in, 2 out]
        n154 = property on="Camera:Exposure" class="DigNum (strict)"("Value"=w319) -> ()  [unwired: 2 in, 2 out]
        n155 = call <vilib>:"Add State(s) to Queue__jki_lib_state_machine.vi"("State(s) in (\"\")"=w329) -> ("States Out"=w328:string)  [unwired: 14 in]
      }
      frame "Camera: Destroy" {
        # "Your code here.\n(You can make a copy of, or modify, this frame)"
        n156 = flat-sequence {
          tunnel: w333 -> [w339]
          tunnel: [w338] -> w331
          tunnel: w331 -> [w342]
          tunnel: [w342] -> w330
          tunnel: w334 -> [w345]
          tunnel: [w343] -> w332
          tunnel: w330 -> [w344]
          frame #0 {
            n157 = property on="Camera:Status" class="Bool (strict)"(error in=w339, "Val(Sgnl)"=FALSE ("Value (Signaling)")) -> (error out=w338:errorcluster)  [unwired: 1 in, 1 out]
          }
          frame #1 {
            n158 = Wait (ms)(milliseconds to wait=u32 1000) -> ()  [unwired: 1 out]
          }
          frame #2 {
            n159 = call-dynamic "Disconnect.vi"("error in (no error)"=w344, "NI Vision Camera Device in"=w345) -> ("error out"=w343:errorcluster)  [unwired: 8 in, 1 out]
          }
        }
        n160 = local read "Camera"() -> (w334:refnum<class "NI Vision Camera Device.lvclass">)
        n161 = call <vilib>:"Add State(s) to Queue__jki_lib_state_machine.vi"("State(s) in (\"\")"=w337) -> ("States Out"=w336:string)  [unwired: 14 in]
      }
      frame "Camera: Error" {
        # "Your code here.\n(You can make a copy of, or modify, this frame)"
        n162 = call <vilib>:"Add State(s) to Queue__jki_lib_state_machine.vi"("State(s) in (\"\")"=w349) -> ("States Out"=w348:string)  [unwired: 14 in]
      }
      frame "---------- Experiment ----------" {
        # "Template Separator\n(You can make a copy of, or modify, this frame)"
        n163 = call <vilib>:"Add State(s) to Queue__jki_lib_state_machine.vi"("State(s) in (\"\")"=w353) -> ("States Out"=w352:string)  [unwired: 14 in]
      }
      frame "Experiment: Start" {
        # "Your code here.\n(You can make a copy of, or modify, this frame)"
        n164 = local write "Exp:Count"(u64 0 ("Exp:Count")) -> ()
        n165 = call <vilib>:"Add State(s) to Queue__jki_lib_state_machine.vi"("State(s) in (\"\")"=w358) -> ("States Out"=w357:string)  [unwired: 14 in]
      }
      frame "Experiment: Abort" {
        # "Your code here.\n(You can make a copy of, or modify, this frame)"
        n166 = local write "Exp:Cont"(FALSE ("Exp:Cont")) -> ()
        n167 = local write "Exp:Start"(FALSE ("Exp:Start")) -> ()
        n168 = call <vilib>:"Add State(s) to Queue__jki_lib_state_machine.vi"("State(s) in (\"\")"=w364) -> ("States Out"=w363:string)  [unwired: 14 in]
      }
      frame "Experiment: Continue" {
        # "Your code here.\n(You can make a copy of, or modify, this frame)"
        n169 = call <vilib>:"Add State(s) to Queue__jki_lib_state_machine.vi"("State(s) in (\"\")"=w368) -> ("States Out"=w367:string)  [unwired: 14 in]
      }
      frame "Experiment: Save" {
        # "Check length of suffix"
        # "Generate filename from time"
        n170 = Get Date/Time In Seconds() -> (seconds since 1Jan1904=w381:timestamp)
        n171 = local read "Camera:FrameCount"() -> (w374:u64)
        n172 = String Length(string="Suffix") -> (length=w383:i32)
        n173 = Format Date/Time String(time format string (%c)="%Y%m%d_%H%M%S", seconds (now)=w381) -> (date/time string=w379:string)  [unwired: 1 in]
        n174 = Equal To 0?(x=w383) -> (x = 0?=w380:bool)
        n175 = case shown="True" w380 {
          tunnel: w379 -> [w393 w394]
          tunnel: [w390 w394] -> w377
          tunnel: "Suffix" -> [w391 _]
          frame False {
            n176 = Concatenate Strings(w393, "_" ("string"), w391) -> (w390:string)
          }
          frame True {
          }
        }
        n177 = Number To Decimal String(number=w374) -> (decimal integer string=w375:string)  [unwired: 1 in]
        n178 = invoke on="Avg" class="IntGraph (strict)" method="Get Image"("image depth"=16 ("Image Depth")) -> ("image data"=w371:T7)  [unwired: 5 in, 5 out]
        n179 = local read "Camera:Sum"() -> (w384:u64[][])
        n180 = local read "App:Basepath"() -> (w372:path)
        n181 = Concatenate Strings(w377, "_" ("string"), w375) -> (w370:string)
        n182 = Divide(x=w384, y=w374) -> (x/y=w373:dbl[][])
        n183 = call "[CS] [Frame] Save to Image File.vi"("image data"=w371, "Name"=w370, "base path"=w372) -> ()  [unwired: 9 in]
        n184 = call "[CS] [Frame] Save to Davis File.vi"("array"=w373, "Name"=w370, "base path"=w372) -> ()  [unwired: 9 in]
        n185 = call "[CS] [Frame] Save to File.vi"("array"=w373, "Name"=w370, "base path"=w372) -> ()  [unwired: 9 in]
        n186 = call <vilib>:"Add State(s) to Queue__jki_lib_state_machine.vi"("State(s) in (\"\")"=w389, "State(s) at Back (\"\")"="UI: Cursor Set >> Idle" ("State(s) at Back (\"\")")) -> ("States Out"=w388:string)  [unwired: 13 in]
      }
      frame "Experiment: Stop" {
        # "Your code here.\n(You can make a copy of, or modify, this frame)"
        n187 = call <vilib>:"Add State(s) to Queue__jki_lib_state_machine.vi"("State(s) in (\"\")"=w399, "State(s) at Back (\"\")"="Experiment: Save" ("State(s) at Back (\"\")")) -> ("States Out"=w398:string)  [unwired: 13 in]
      }
    }
  }
